vi "switch.vi"() -> ()   [LabVIEW 2010]
uses:
  <vilib>/DAQmx/write.llb/DAQmx Write (Digital 1D Bool 1Chan 1Samp).vi
  <vilib>/DAQmx/create/channels.llb/DAQmx Create Channel (DO-Digital Output).vi
  <vilib>/daqmx/miscellaneous.llb/DAQmx Fill In Error Info.vi
panel:
  in  "Boolean 2":bool
  in  "Boolean1":bool
  in  "Boolean0":bool
  out "concatenated string":string
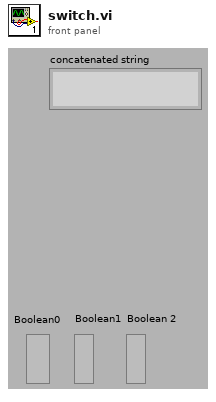
[diagram p1: front panel]
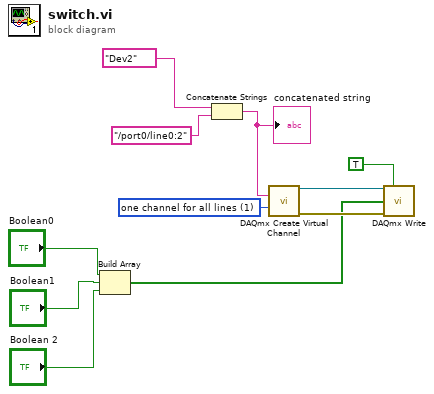
[diagram p0: block diagram]
diagram:
  w1 = 1 items=["one channel for each line", "one channel for all lines"] ("line grouping")
  n1 = Build Array("Boolean0", "Boolean1", "Boolean 2") -> (w2:bool[])
  n2 = Concatenate Strings(tag "Dev2" ("string"), "/port0/line0:2") -> (w8:string)
  "concatenated string" <- w8
  n3 = call-poly <vilib>:"DAQmx Create Virtual Channel.vi"("lines"=w8, "line grouping"=w1) -> ("task out"=w11:refnum<k21>, "error out"=w10:errorcluster)  [unwired: 12 in]
  n4 = call-poly <vilib>:"DAQmx Write.vi"("task/channels in"=w11, "auto start"=TRUE, "data"=w2, "error in"=w10) -> ()  [unwired: 9 in, 3 out]
